vi "AlliGator Store Cursor-defined Head & Tail Fractions.vi"(8 "error in (no error)":errorcluster, 11 "Selected Plot Info":T1={"Multiplot XY Graph"=refnum, "Mouse Coordinates"={"Horizontal"=0, "Vertical"=0}, "Plot Index"=-1}) -> (0 "Error Out":errorcluster, 2 "Message":string)   [LabVIEW 2021, in "AlliGator Decay Analysis.lvlib" / "AlliGator Decay Preprocessing.lvlib"]
doc: "Sets the head and tail fractions for decay extrapolation based on the corresponding cursor locations.\n\nIf one cursor is missing, the current fraction is preserved."
uses:
  AlliGator Decay Preprocessing.lvlib
  Graphs/XY Graph/XY Graph Selected Plot Info.ctl
  Graphs/XY Graph/XY Graph Refnum.ctl
  <vilib>/Utility/miscctls.llb/LVPoint32TypeDef.ctl
  AlliGator Settings List.ctl
  AlliGator Settings Event.ctl
  AlliGator Settings Window Messages.ctl
  Variant/Variant to Data/Variant to DBL.vi
  Variant/Variant to Data/Variant to Boolean.vi
  AlliGator Settings.lvlib
  Variant/Variant to Data/Variant to Data.lvlib
  Graphs/XY Graph/XY Graph Add-Ons.lvlib
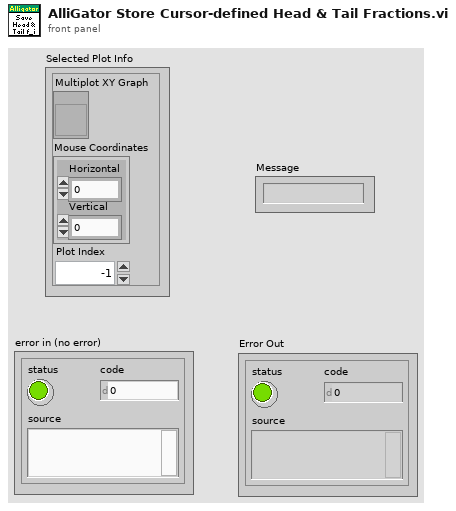
[diagram p1: front panel]
types:
  T1 = typedef "XY Graph Add-Ons.lvlib/XY Graph Selected Plot Info.ctl" = cluster{"Multiplot XY Graph":T2, "Mouse Coordinates":T3, "Plot Index":i32}
  T2 = typedef "XY Graph Add-Ons.lvlib/XY Graph Refnum.ctl" = refnum<vi>
  T3 = typedef "LVPoint32TypeDef.ctl" = cluster{"Horizontal":i32, "Vertical":i32}
  T4 = typedef "AlliGator Settings.lvlib/AlliGator Settings List.ctl" = enum16{"GUI:Visible Settings Tab", "GUI:Last Run Version", "Source Image:Use Image Histogram for Contrast", "Source Image:Low Count Pixels Rejection Options", "Source Image:High Count Pixels Rejection Options", "Source Image:Use Image Brightness", "Source Image:Blend Overlay with Image Background", "Source Image:Use Fixed ROI Diameter", "Source Image:ROI Diameter", "Source Image:ROI Center Color", "Source Image:Peak Threshold", "Source Image:Intensity Threshold", "Source Image:Image Binning Options", "Source Image:Image Smoothing Options", "Source Image:Image Histogram Active", "Source Image:Invert Binary Mask", "Source Image:Hot Pixel Removal", "Source Image:Overlay Analyzed ROI Center", "Source Image:Auto-Adjust Contrast", "Source Image:Histogram Lower Percentile", "Source Image:Histogram Upper Percentile", "Source Image:Save Source Image", "Source Image:Scale Bar Options", "Source Image:Image Resolution (Pixel Size)", "Source Image:Flatfield Correction", "Source Image:Show Dead Left Columns Correction", "Source Image:Dead Left Columns Correction", "Source Image:Image Pre-Processing Operations Order", "Data Information:Gate Width", "Data Information:Nanotime Gate Separation", "Data Information:Macrotime Gate Separation", "Data Information:Gate Step", "Data Information:# Gates", "Data Information:Gate Image Exposure", "Data Information:Gate Image Integration", "Data Information:Gates to Skip", "Data Information:Gates to Keep", "Data Information:Define Gates to", "Data Information:Channel Name", "Data Information:Available Channel Names", "Data Information:Channel Arithmetic", "Data Information:Background File Subtraction", "Data Information:Background File", "Data Information:Background Scaling Factor", "Data Information:Background Pile-up Correction", "Data Information:Background Pixel Well Capacity", "Data Information:Laser Period", "Data Information:SYNC Period", "Data Information:Pile-up Correction", "Data Information:Pixel Well Capacity", "Data Information:Dataset Scaling Factor", "Fluorescence Decay_Decay Pre-Processing:Reverse Gates", "Fluorescence Decay_Decay Pre-Processing:Verbose Decay Pre-Processing", "Fluorescence Decay_Decay Pre-Processing:Use Decay Pre-Processing", "Fluorescence Decay_Decay Pre-Processing:Background Subtraction", "Fluorescence Decay_Decay Pre-Processing:Background Definition Range", "Fluorescence Decay_Decay Pre-Processing:Baseline Subtraction Method", "Fluorescence Decay_Decay Pre-Processing:Decay Pre-Processing Operations Order", "Fluorescence Decay_Decay Pre-Processing:Smoothing Parameter", "Fluorescence Decay_Decay Pre-Processing:Shift Decay", "Fluorescence Decay_Decay Pre-Processing:Decay Shift Parameters", "Fluorescence Decay_Decay Pre-Processing:Fold Decay", "Fluorescence Decay_Decay Pre-Processing:# Folds", "Fluorescence Decay_Decay Pre-Processing:1-Normalize Decay", "Fluorescence Decay_Decay Pre-Processing:[0-1]-Normalize Decay", "Fluorescence Decay_Decay Pre-Processing:Smoothen Decay", "Fluorescence Decay_Decay Pre-Processing:Extrapolate Decay", "Fluorescence Decay_Decay Pre-Processing:Use Periodicity", "Fluorescence Decay_Decay Pre-Processing:Use Cursors", "Fluorescence Decay_Decay Pre-Processing:Tail Fraction", "Fluorescence Decay_Decay Pre-Processing:Head Fraction", "Fluorescence Decay_Decay Pre-Processing:Additional Points", "Fluorescence Decay_Decay Pre-Processing:Straighten Decay", "Fluorescence Decay_Decay Pre-Processing:Constant Background", "Fluorescence Decay_Decay Pre-Processing:Pixel-Normalize Decay", "Fluorescence Decay_Advanced Analysis:Extract IRF instead of Decay", "Fluorescence Decay_Advanced Analysis:IRF Extraction Options", "Fluorescence Decay_Advanced Analysis:IRF Optimization Options", "Fluorescence Decay_Advanced Analysis:Square Pulse Options", "Fluorescence Decay_Advanced Analysis:IRF Order", "Fluorescence Decay_Advanced Analysis:IRF Time Constants", "Fluorescence Decay_Advanced Analysis:Wavelet Analysis Options", "Fluorescence Decay_Advanced Analysis:Average Lifetime Options", "Fluorescence Decay_Fit Options:Fit Options", "Fluorescence Decay_Fit Options:Use Legacy Fitting Approach", "Fluorescence Decay_Fit Options:Use Data Information Laser Period", "Fluorescence Decay_Fit Parameters:Displayed Fit Parameters", "Fluorescence Decay_Fit Parameters:Fit Parameter Constraints", "Fluorescence Decay_Fit Parameters:Export Tabulated Results", "Fluorescence Decay_Fit Parameters:MLE Baseline Offset Type", "Fluorescence Decay_Fit Parameters:MLE Baseline Offset", "Fluorescence Decay_Fit Parameters:Guess Parameter Names", "Fluorescence Decay_Fit Parameters:Guess Parameter Values", "Fluorescence Decay_Fit Parameters:Guess Parameters Options", "Fluorescence Decay_Styles:Show Last Decay Only", "Fluorescence Decay_Styles:Decay Graph Color Array", "Fluorescence Decay:Decay Graph Active", "Fluorescence Decay Statistics:Min Peak Value", "Fluorescence Decay Statistics:Reject Low Decay Peak Pixels", "Fluorescence Decay Statistics:Reject High Decay Peak Pixels", "Fluorescence Decay Statistics:Max Peak Value", "Time Traces:Use File Timestamp", "Time Traces:Time Step", "Time Traces:Use Intensity Correction File", "Time Traces:Intensity Correction File", "Phasor Plot:Phasor Plot Smoothing Options", "Phasor Plot:Phasor Plot Size", "Phasor Plot:Phasor Plot Graphics Options", "Phasor Plot:Cumulative Phasor Plot", "Phasor Plot:Use Phasor Brightness", "Phasor Plot:Blend Overlay with Phasor Background", "Phasor Plot:Save Phasor Plot", "Phasor Plot:Show References", "Phasor Plot:Phasor Ratio Decay Range", "Phasor Plot:Exponential Fading", "Phasor Plot:Phasor Ratio Reference Colors", "Phasor Plot:Reference Radius", "Phasor Plot:Show Color Map Vertices", "Phasor Plot:Phasor Plot Active", "Phasor Plot:Phasor Ratio Color Map Type", "Phasor Plot:Phasor Ratio Color Map", "Phasor Plot:Phasor Ratio Display Range", "Phasor Plot:Selected Image ROI(s)", "Phasor Plot:All Image ROIs", "Phasor Plot:Selected Phasor Plot ROI(s)", "Phasor Plot:All Phasor Plot ROIs", "Phasor Plot:Phasor Ratio Color-Coded Quantity", "Phasor Plot:Store Phasor Harmonics", "Phasor Plot:Draw Reference Segment", "Phasor Plot:User-Defined Quantity", "Phasor Graph:Phasor Frequency", "Phasor Graph:Phasor Ratio Type", "Phasor Graph:Pixel-level Phasor Computation", "Phasor Graph:Save Phasor Graph", "Phasor Graph:Phasor Graph Active", "Phasor Graph:Phasor SDV Options", "Phasor Calibration:Use Backup Calibration if needed", "Phasor Graph:Define Shortest Lifetime as", "Phasor Calibration:Backup Calibration Type", "Phasor Calibration:Calibration Type", "Phasor Calibration:Calibration Lifetime", "Phasor Calibration:Calibration Map Algorithm", "Single-Exponential Phasor Locus (SEPL):Gate Parameters", "Single-Exponential Phasor Locus (SEPL):User-defined Gate", "Single-Exponential Phasor Locus (SEPL):User-defined IRF", "Single-Exponential Phasor Locus (SEPL):Phasor Parameters", "Single-Exponential Phasor Locus (SEPL):Decay & IRF Parameters", "Single-Exponential Phasor Locus (SEPL):Display Parameters", "Lifetime Analysis:Decay Analysis Parameters", "Lifetime Analysis:Lifetime Map Active", "Plugins:Python Settings", "Miscellaneous:Verbose Mode", "Miscellaneous:Beep after Script", "Miscellaneous:Saved Image File Format", "Miscellaneous:Exported Gate Image Settings", "Miscellaneous:Include Loading in Timing", "Miscellaneous:Verbose Settings Mode", "Miscellaneous:Histogram Options", "Miscellaneous:Beep on Error", "Miscellaneous:# Logical Processors Used", "Miscellaneous:ROI Description Max Characters", "Miscellaneous:Verbose Error Mode", "Miscellaneous:Transparent Mask Color"}
  T5 = typedef "AlliGator Settings.lvlib/AlliGator Settings Event.ctl" = cluster{"AlliGator Settings Message":T6, "Sender":string, "Control Label":string, "Data":variant}
  T6 = typedef "AlliGator Settings.lvlib/AlliGator Settings Window Messages.ctl" = enum16{"Idle", "Subscribe", "Unsubscribe", "Refresh Parameter", "Refresh All Parameters", "Quit"}
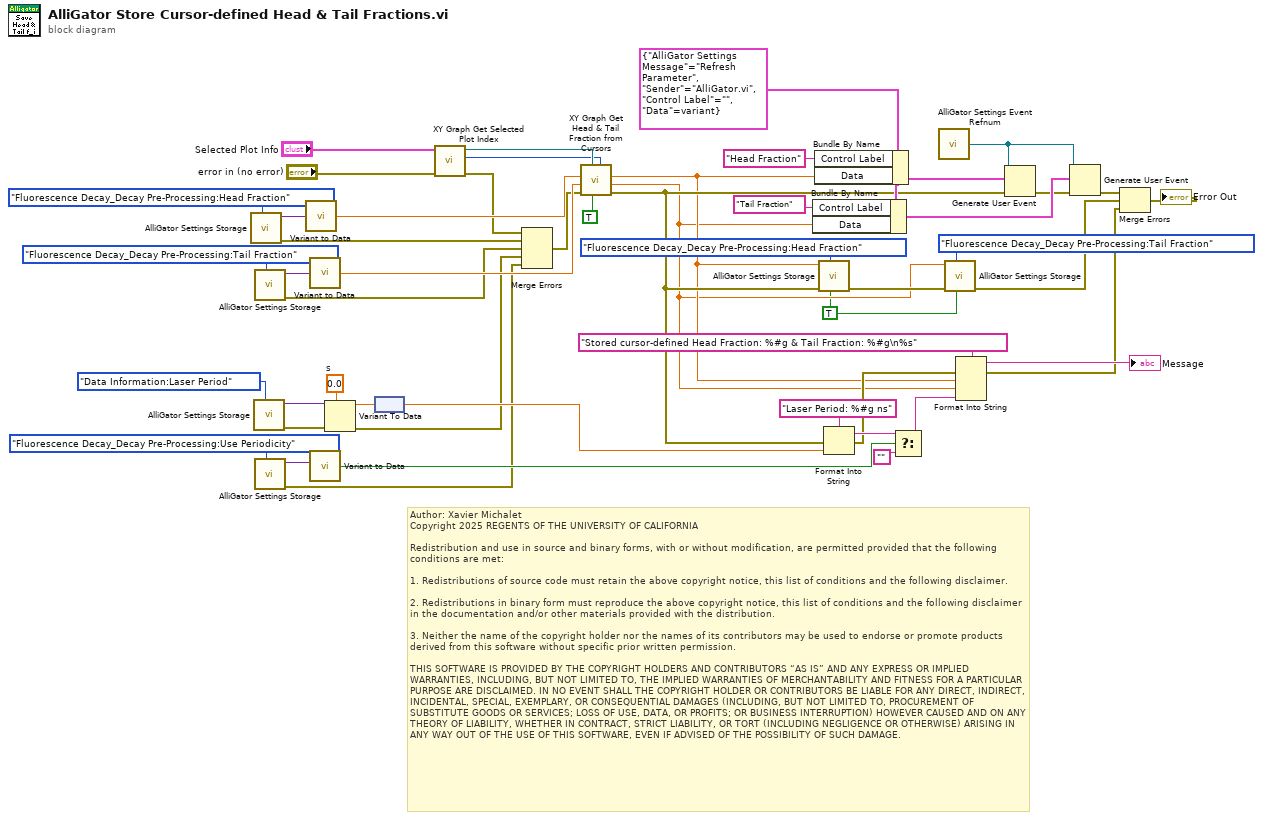
[diagram p0: block diagram]
diagram:
  w9 = TRUE ("Get(F)/Set")
  w29 = T5 {"AlliGator Settings Message"=enum."Refresh Parameter", "Sender"="AlliGator.vi", "Control Label"="", "Data"=variant} ("AlliGator Settings Event")
  w44 = dbl[unit] 0.0  # s
  # "Author: Xavier Michalet\nCopyright 2025 REGENTS OF THE UNIVERSITY OF CALIFORNIA\n\nRedistribution and use in source and binary forms, with or without modification, are permitted provided that the following conditions are met:\n\n1. Redistributions of source code must retain the above copyright notice, this list of conditions and the following disclaimer.\n\n2. Redistributions in binary form must reproduce the above copyright notice, this list of conditions and the following disclaimer in the documentation and/or other materials provided with the distribution.\n\n3. Neither the name of the copyright holder nor the names of its contributors may be used to endorse or promote products derived from this software without specific prior written permission.\n\nTHIS SOFTWARE IS PROVIDED BY THE COPYRIGHT HOLDERS AND CONTRIBUTORS “AS IS” AND ANY EXPRESS OR IMPLIED WARRANTIES, INCLUDING, BUT NOT LIMITED TO, THE IMPLIED WARRANTIES OF MERCHANTABILITY AND FITNESS FOR A PARTICULAR PURPOSE ARE DISCLAIMED. IN NO EVENT SHALL THE COPYRIGHT HOLDER OR CONTRIBUTORS BE LIABLE FOR ANY DIRECT, INDIRECT, INCIDENTAL, SPECIAL, EXEMPLARY, OR CONSEQUENTIAL DAMAGES (INCLUDING, BUT NOT LIMITED TO, PROCUREMENT OF SUBSTITUTE GOODS OR SERVICES; LOSS OF USE, DATA, OR PROFITS; OR BUSINESS INTERRUPTION) HOWEVER CAUSED AND ON ANY THEORY OF LIABILITY, WHETHER IN CONTRACT, STRICT LIABILITY, OR TORT (INCLUDING NEGLIGENCE OR OTHERWISE) ARISING IN ANY WAY OUT OF THE USE OF THIS SOFTWARE, EVEN IF ADVISED OF THE POSSIBILITY OF SUCH DAMAGE."
  n1 = call "AlliGator Settings Storage.vi"("AlliGator Settings List"=AlliGator_Settings_List."Fluorescence Decay_Decay Pre-Processing:Head Fraction") -> ("Error Out"=w21:errorcluster, "Variant Data out"=w41:variant)  [unwired: 9 in]
  n2 = call "AlliGator Settings Storage.vi"("AlliGator Settings List"=AlliGator_Settings_List."Data Information:Laser Period") -> ("Error Out"=w45:errorcluster, "Variant Data out"=w46:variant)  [unwired: 9 in]
  n3 = call "AlliGator Settings Storage.vi"("AlliGator Settings List"=AlliGator_Settings_List."Fluorescence Decay_Decay Pre-Processing:Tail Fraction") -> ("Error Out"=w20:errorcluster, "Variant Data out"=w50:variant)  [unwired: 9 in]
  n4 = call "AlliGator Settings Storage.vi"("AlliGator Settings List"=AlliGator_Settings_List."Fluorescence Decay_Decay Pre-Processing:Use Periodicity") -> ("Error Out"=w18:errorcluster, "Variant Data out"=w49:variant)  [unwired: 9 in]
  n5 = call-poly "Variant to Data.vi"("Variant"=w41) -> ("Value"=w39:dbl)  [unwired: 8 in]
  n6 = call-poly "Variant to Data.vi"("Variant"=w50) -> ("Value"=w42:dbl)  [unwired: 8 in]
  n7 = call-poly "Variant to Data.vi"("Variant"=w49) -> ("Value"=w35:bool)  [unwired: 8 in]
  n8 = Variant To Data(error in=w45, type=w44, Variant=w46) -> (data=w43:dbl[unit], error out=w19:errorcluster)
  n9 = node(w43) -> (w32:dbl)
  n10 = call "XY Graph Get Selected Plot Index.vi"("error in (no error)"="error in (no error)", "Selected Plot Info"="Selected Plot Info") -> ("error out"=w1:errorcluster, "Plot at Coordinates"=w2:i32, "XYGraph out"=w3:T2)  [unwired: 6 in, 1 out]
  n11 = Merge Errors(w1, w21, w20, w19, w18) -> (w22:errorcluster)
  n12 = call "XY Graph Get Head & Tail Fraction from Cursors.vi"("Active Plot Index"=w2, "Use Cursors"=TRUE, "XYGraph in"=w3, "error in (no error)"=w22, "Tail Fraction"=w42, "Head Fraction"=w39) -> ("error out"=w15:errorcluster, "Tail Fraction"=w11:dbl, "Head Fraction"=w13:dbl)  [unwired: 1 in, 2 out]
  n13 = Bundle By Name(cluster=w29, "Control Label"="Tail Fraction", "Data"=w11) -> (w26:T5)
  n14 = Bundle By Name(cluster=w29, "Control Label"="Head Fraction", "Data"=w13) -> (w28:T5)
  n15 = call "AlliGator Settings Storage.vi"("Get(F)/Set"=w9, "AlliGator Settings List"=AlliGator_Settings_List."Fluorescence Decay_Decay Pre-Processing:Head Fraction", "Error In"=w15, "Variant Data in"=w13) -> ("Error Out"=w12:errorcluster)  [unwired: 6 in, 1 out]
  n16 = Format Into String(format string="Laser Period: %#g ns", error in=w15, w32) -> (resulting string=w33:string, error out=w17:errorcluster)  [unwired: 1 in]
  n17 = Select(t=w33, s=w35, f="") -> (s? t:f=w36:string)
  n18 = call "AlliGator Settings Event Refnum.vi"() -> ("AlliGator Settings Event Refnum"=w27:refnum<user-event>)  [unwired: 8 in, 1 out]
  n19 = call "AlliGator Settings Storage.vi"("Get(F)/Set"=w9, "AlliGator Settings List"=AlliGator_Settings_List."Fluorescence Decay_Decay Pre-Processing:Tail Fraction", "Error In"=w12, "Variant Data in"=w11) -> ("Error Out"=w8:errorcluster)  [unwired: 6 in, 1 out]
  n20 = Format Into String(format string="Stored cursor-defined Head Fraction: %#g & Tail Fraction: %#g\n%s", error in=w17, w13, w11, w36) -> (resulting string=→"Message":string, error out=w6:errorcluster)  [unwired: 1 in]
  n21 = Generate User Event(user event=w27, event data cluster=w28, error in=w15) -> (error out=w25:errorcluster)  [unwired: 1 in, 1 out]
  n22 = Generate User Event(user event=w27, event data cluster=w26, error in=w25) -> (error out=w24:errorcluster)  [unwired: 1 in, 1 out]
  n23 = Merge Errors(w24, w8, w6) -> (→"Error Out":errorcluster)
